vi "oa_Average DC Value.vi"(7 "reset?":bool=TRUE, 8 "error in":errorcluster, 11 "value in":dbl[](array[numeric])) -> (0 "error out":errorcluster, 3 "value":dbl)   [LabVIEW 2017, in "SoundVib_RefDataProcess.lvlib"]
uses:
  <vilib>/addons/Sound and Vibration/Order Analysis/Referece Data Processing/SoundVib_RefDataProcess.lvlib
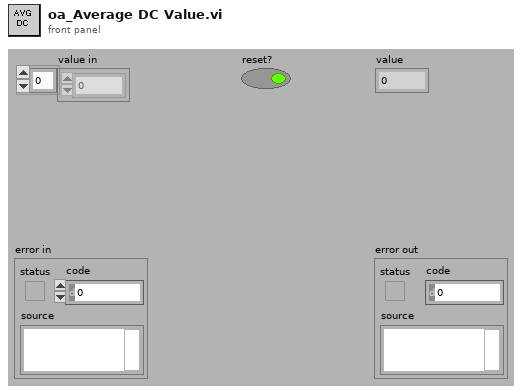
[diagram p1: front panel]
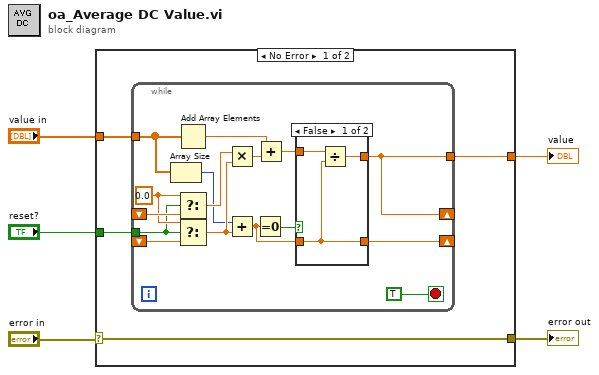
[diagram p0: block diagram]
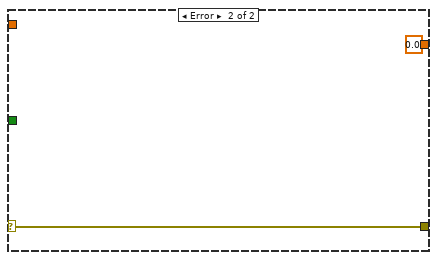
[diagram p3: hidden frame]
diagram:
  n1 = case shown="No Error" "error in" {
    selector: "error in" -> [w8 w32]
    tunnel: [w8 w32] -> w4
    tunnel: "reset?" -> [w9 _]
    tunnel: "value in" -> [w7 _]
    tunnel: [w6 0.0] -> w1
    frame No Error {
      n2 = while {
        shift-right: [w13] -> _
        shift-left: _ -> [w24]
        shift-right: [w12] -> _
        shift-left: _ -> [w23]
        tunnel: w9 -> [w21]
        tunnel: w7 -> [w15]
        tunnel: [w13] -> w6
        stop <- TRUE stop-if-true
        w22 = 0.0 ("t")
        n3 = Array Size(array=w15) -> (size(s)=w14:i32)
        n4 = Add Array Elements(numeric array=w15) -> (sum=w17:dbl)
        n5 = Select(t=w22, s=w21, f=w24) -> (s? t:f=w20:dbl)
        n6 = Select(t=w22, s=w21, f=w23) -> (s? t:f=w16:dbl)
        n7 = Multiply(x=w20, y=w16) -> (x*y=w19:dbl)
        n8 = Add(x=w14, y=w16) -> (x+y=w10:dbl)
        n9 = Equal To 0?(x=w10) -> (x = 0?=w11:bool)
        n10 = Add(x=w17, y=w19) -> (x+y=w18:dbl)
        n11 = case shown="False" w11 {
          tunnel: w18 -> [w28 w30]
          tunnel: [w27 w30] -> w13
          tunnel: [w26 w29] -> w12
          tunnel: w10 -> [w26 w29]
          frame False {
            n12 = Divide(x=w28, y=w26) -> (x/y=w27:dbl)
          }
          frame True {
          }
        }
      }
    }
    frame Error {
    }
  }
  "error out" <- w4
  "value" <- w1
